vi "FTW-CodeGen-Initialize.vi"(5 "XRef":refnum<vi>) -> (4 "State Out":T1)   [LabVIEW 2014, in "FTW-SQLite-Fetch.xnode"]
uses:
  FTW-SQLite-Fetch.xnode
  FTW-CodeGen-State.ctl
panel:
  # "Inputs"
  # "Outputs"
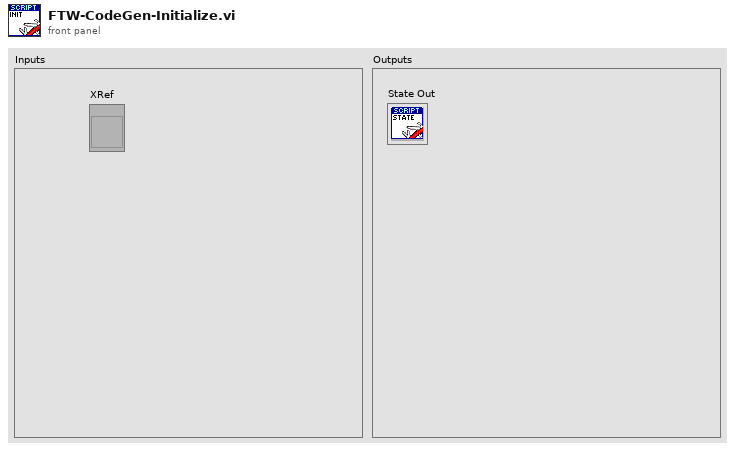
[diagram p1: front panel]
types:
  T1 = typedef "FTW-SQLite-Fetch.xnode/FTW-CodeGen-State.ctl" = cluster{"Dummy":i32}
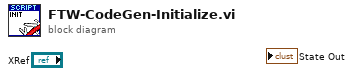
[diagram p0: block diagram]
diagram:
